vi "Apply.vi"(8 "Error In":errorcluster, 11 "object in":refnum<class "Continuous Waveform Acq CFG.lvclass">) -> (0 "Error Out":errorcluster, 3 "object out":refnum<class "Continuous Waveform Acq CFG.lvclass">)   [LabVIEW 2023, in "Continuous Waveform Acq CFG.lvclass"]
uses:
  Continuous Waveform Acq CFG.lvclass
  Continuous Waveform Acq CFG.lvclass/Continuous Waveform Acq CFG.ctl
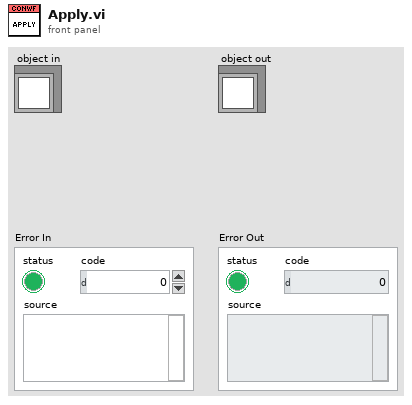
[diagram p1: front panel]
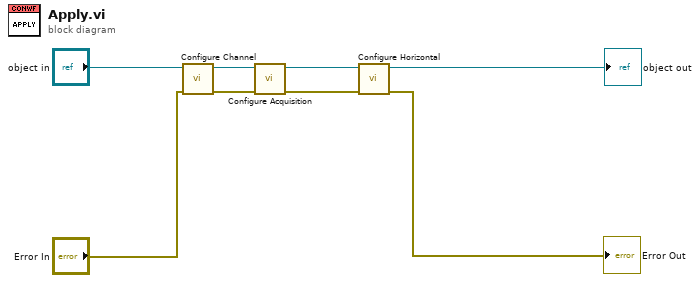
[diagram p0: block diagram]
diagram:
  n1 = call-dynamic "Configure Channel.vi"("error in"="Error In", "Continuous Waveform Acq CFG in"="object in") -> ("error out"=w6:errorcluster, "Continuous Waveform Acq CFG out"=w4:refnum<class "Continuous Waveform Acq CFG.lvclass">)  [unwired: 8 in]
  n2 = call-dynamic "Configure Acquisition.vi"("error in"=w6, "Continuous Waveform Acq CFG in"=w4) -> ("error out"=w5:errorcluster, "Continuous Waveform Acq CFG out"=w2:refnum<class "Continuous Waveform Acq CFG.lvclass">)  [unwired: 8 in]
  n3 = call "Configure Horizontal.vi"("error in (no error)"=w5, "Continuous Waveform Acq CFG in"=w2) -> ("error out"=→"Error Out":errorcluster, "Continuous Waveform Acq CFG out"=→"object out":refnum<class "Continuous Waveform Acq CFG.lvclass">)  [unwired: 8 in]
